vi "SSD1306_SaveImages2File.vi"(1 "vi name":string) -> (0 "file name":string)   [LabVIEW 2014, in "QwaveSys_Interface.lvlib"]
uses:
  QwaveSys_Interface.lvlib
  <vilib>/Utility/traverseref.llb/TRef TravTarget.ctl
  <vilib>/Utility/sysdir.llb/System Directory Type.ctl
  <vilib>/Utility/traverseref.llb/VI Scripting - Traverse.lvlib
panel:
  out "error out":errorcluster
  out "Images":string
  out "found":bool
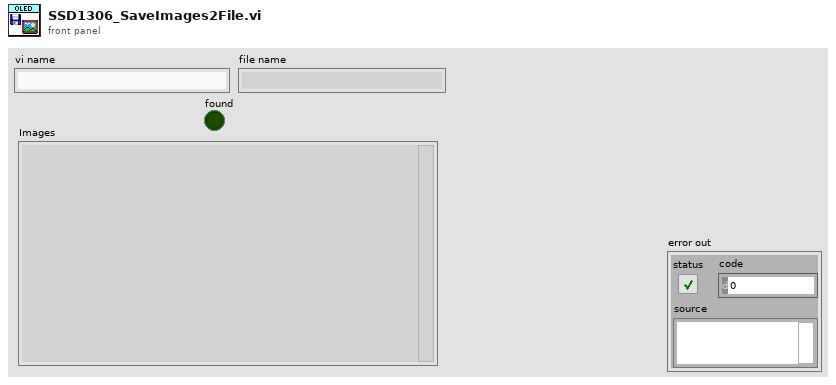
[diagram p1: front panel]
types:
  T1 = typedef "System Directory Type.ctl" = i32
  T2 = typedef "TRef TravTarget.ctl" = enum16{"FP", "BD", "Other"}
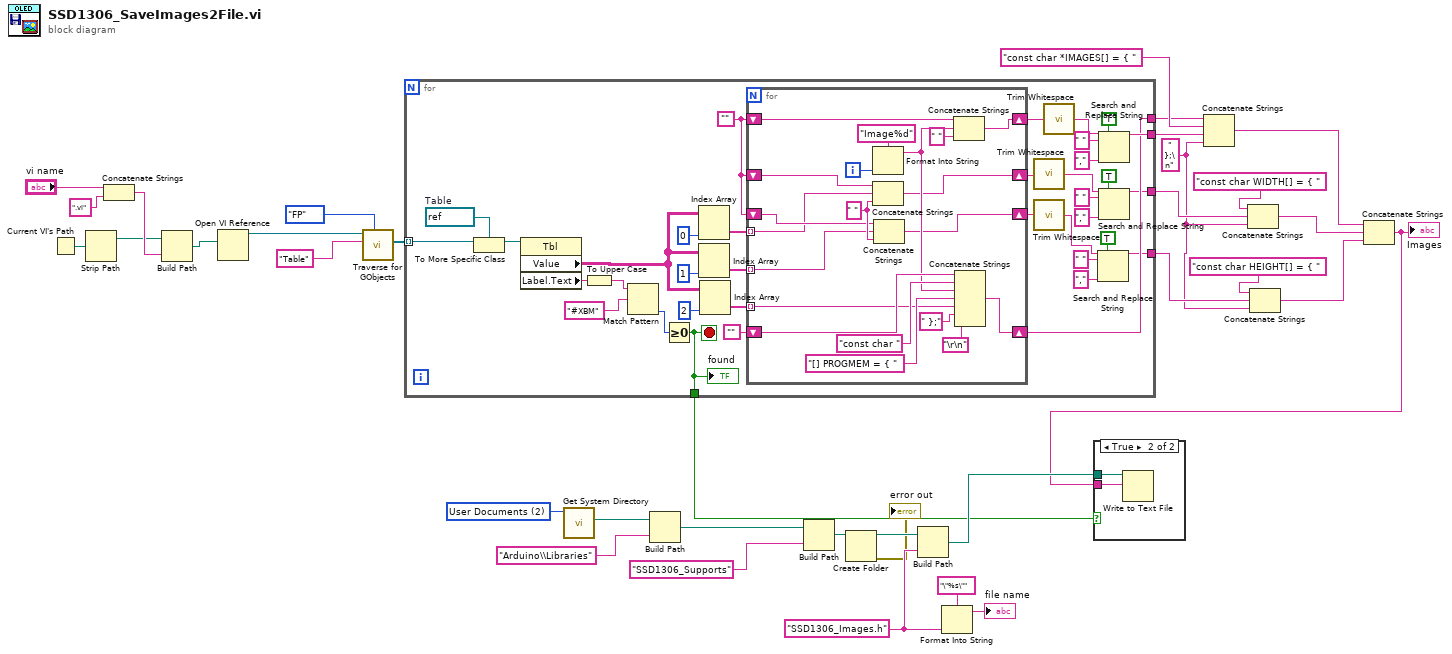
[diagram p0: block diagram]
diagram:
  w5 = " };\n" ("string")
  w25 = T1 2 items=["User Home"=0, "User Desktop"=1, "User Documents"=2, "User Application Data"=3, "User Preferences"=4, "User Temporary"=5, "Public Documents"=6, "Public Application Data"=7, "Public Preferences"=8, "Public Cache"=13, "System Core Libraries"=9, "System Installed Libraries"=10, "Application Files"=11, "Boot Volume Root"=12] ("system directory type")
  w20 = "SSD1306_Images.h" ("string")
  n1 = Current VI's Path() -> (path=w29:path)
  n2 = Strip Path(path=w29) -> (stripped path=w28:path)  [unwired: 1 out]
  n3 = Concatenate Strings("vi name", ".vi" ("string")) -> (w30:string)
  n4 = Build Path(base path=w28, name or relative path=w30) -> (appended path=w26:path)
  n5 = Open VI Reference(vi path=w26) -> (vi reference=w35:refnum<vi>)  [unwired: 5 in, 1 out]
  n6 = call <vilib>:"Traverse for GObjects.vi"("Traverse Target"=TRef_TravTarget."FP", "Class Name"="Table", "VI Refnum"=w35) -> ("References"=w33:refnum<vi>[])  [unwired: 5 in, 3 out]
  n7 = for {
    tunnel: w33 -> [w70] mode=indexing
    tunnel: [w61] -> w15
    tunnel: [w56] -> w13
    tunnel: [w54] -> w11
    tunnel: [w37] -> w6
    tunnel: [w36] -> w7
    stop <- w61 stop-if-true
    w48 = ""
    w69 = refnum<vi> refnum  # Table
    n8 = To More Specific Class(target class=w69, reference=w70) -> (specific class reference=w71:refnum<vi>)  [unwired: 1 in, 1 out]
    n9 = property class="Tbl"(reference=w71) -> ("Value"=w51:string[][], "Label.Text"=w68:string)  [unwired: 1 in, 2 out]
    n10 = To Upper Case(1:w68) -> (0:w67:string)
    n11 = Match Pattern(string=w67, regular expression="#XBM") -> (offset past match=w66:i32)  [unwired: 1 in, 3 out]
    n12 = Greater Or Equal To 0?(x=w66) -> (x >= 0?=w61:bool)
    "found" <- w61
    n13 = Index Array(array=w51, index (col)=0 ("disabled index (col)")) -> (element=w50:string[])  [unwired: 1 in]
    n14 = Index Array(array=w51, index (col)=1 ("disabled index (col)")) -> (element=w49:string[])  [unwired: 1 in]
    n15 = Index Array(array=w51, index (col)=2 ("disabled index (col)")) -> (element=w63:string[])  [unwired: 1 in]
    n16 = for {
      tunnel: w63 -> [w80] mode=indexing
      shift-right: [w85] -> w54
      shift-left: "" -> [w88]
      shift-right: [w82] -> w60
      shift-left: w48 -> [w84]
      tunnel: w50 -> [w74] mode=indexing
      tunnel: w49 -> [w75] mode=indexing
      shift-right: [w73] -> w47
      shift-left: w48 -> [w77]
      shift-right: [w72] -> w46
      shift-left: w48 -> [w76]
      i -> [w91]
      w78 = " " ("string")
      n17 = Format Into String(format string="Image%d", w91) -> (resulting string=w79:string)  [unwired: 2 in, 1 out]
      n18 = Concatenate Strings(w77, w74, w78) -> (w73:string)
      n19 = Concatenate Strings(w76, w75, w78) -> (w72:string)
      n20 = Concatenate Strings(w84, w79, " " ("string")) -> (w82:string)
      n21 = Concatenate Strings(w88, "const char " ("format string"), w79, "[] PROGMEM = { " ("format string"), w80, " };" ("string"), "\r\n") -> (w85:string)
    }
    n22 = call <vilib>:"Trim Whitespace.vi"("string"=w47) -> ("trimmed string"=w39:string)  [unwired: 1 in]
    n23 = call <vilib>:"Trim Whitespace.vi"("string"=w46) -> ("trimmed string"=w38:string)  [unwired: 1 in]
    n24 = call <vilib>:"Trim Whitespace.vi"("string"=w60) -> ("trimmed string"=w59:string)  [unwired: 1 in]
    n25 = Search and Replace String(replace all?=TRUE ("replace all? (F)"), input string=w38, search string=" ", replace string="," ("replace string (\"\")")) -> (result string=w37:string)  [unwired: 4 in, 3 out]
    n26 = Search and Replace String(replace all?=TRUE ("replace all? (F)"), input string=w59, search string=" ", replace string="," ("replace string (\"\")")) -> (result string=w56:string)  [unwired: 4 in, 3 out]
    n27 = Search and Replace String(replace all?=TRUE ("replace all? (F)"), input string=w39, search string=" ", replace string="," ("replace string (\"\")")) -> (result string=w36:string)  [unwired: 4 in, 3 out]
  }
  n28 = call <vilib>:"Get System Directory.vi"("system directory type"=w25) -> ("system directory"=w23:path)  [unwired: 10 in]
  n29 = Build Path(base path=w23, name or relative path="Arduino\\Libraries") -> (appended path=w16:path)
  n30 = Build Path(base path=w16, name or relative path="SSD1306_Supports") -> (appended path=w19:path)
  n31 = Create Folder(path (use dialog)=w19) -> (created path=w18:path, error out=→"error out":errorcluster)  [unwired: 2 in, 1 out]
  n32 = Build Path(base path=w18, name or relative path=w20) -> (appended path=w17:path)
  n33 = Format Into String(format string="\"%s\"", w20) -> (resulting string=→"file name":string)  [unwired: 2 in, 1 out]
  n34 = Concatenate Strings(w11, "const char *IMAGES[] = { " ("string"), w13, w5) -> (w3:string)
  n35 = Concatenate Strings("const char WIDTH[] = { " ("string"), w7, w5) -> (w2:string)
  n36 = Concatenate Strings("const char HEIGHT[] = { " ("string"), w6, w5) -> (w1:string)
  n37 = Concatenate Strings(w3, w2, w1) -> (w4:string)
  "Images" <- w4
  n38 = case shown="True" w15 {
    tunnel: w4 -> [_ w93]
    tunnel: w17 -> [_ w92]
    frame False {
    }
    frame True {
      n39 = Write to Text File(file (use dialog)=w92, text=w93) -> ()  [unwired: 2 in, 3 out]
    }
  }
